vi "Parser2.vi"(5 "InputString":string="\"arg1 and more arg1\" arg2") -> (2 "Arg2 Out":string, 3 "Arg1 Out":string)   [LabVIEW 2014]
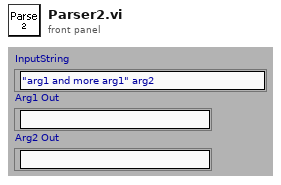
[diagram p1: front panel]
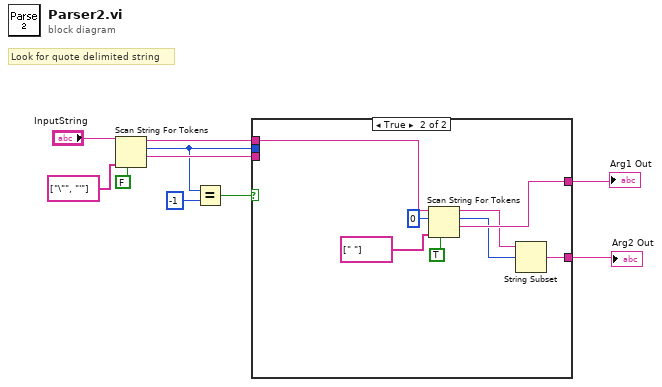
[diagram p0: block diagram]
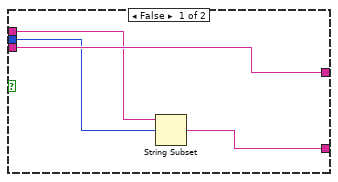
[diagram p2: hidden frame]
diagram:
  # "Look for quote delimited string"
  n1 = Scan String For Tokens(4:FALSE ("use cached delim/oper data? (F)"), 6:string[] ["\"", "'"] ("delimiters (\\s,\\t,\\r,\\n)"), 9:"InputString") -> (1:w4:string, 2:w1:i32, 3:w3:string)  [unwired: 3 in, 1 out]
  n2 = Equal?(x=w1, y=-1) -> (x = y?=w6:bool)
  n3 = case shown="True" w6 {
    tunnel: [w14 w20] -> w5
    tunnel: w4 -> [w14 _]
    tunnel: w3 -> [w13 w19]
    tunnel: [w11 w15] -> w2
    tunnel: w1 -> [w12 _]
    frame False {
      n4 = String Subset(string=w13, offset (0)=w12) -> (substring=w11:string)  [unwired: 1 in]
    }
    frame True {
      n5 = Scan String For Tokens(4:TRUE ("use cached delim/oper data? (F)"), 6:string[] [" "] ("delimiters (\\s,\\t,\\r,\\n)"), 8:0 ("offset"), 9:w19) -> (1:w20:string, 2:w16:i32, 3:w17:string)  [unwired: 2 in, 1 out]
      n6 = String Subset(string=w17, offset (0)=w16) -> (substring=w15:string)  [unwired: 1 in]
    }
  }
  "Arg2 Out" <- w2
  "Arg1 Out" <- w5
